vi "Get Counter Updated Event.vi"(8 "error in (no error)":errorcluster, 11 "Counter in":refnum<class "Counter.lvclass">) -> (0 "error out":errorcluster, 2 "Counter Updated":refnum<user-event>, 3 "Counter out":refnum<class "Counter.lvclass">)   [LabVIEW 2018, in "Counter.lvlib" / "Counter.lvclass"]
uses:
  Counter.lvclass
  Counter.lvclass/Counter.ctl
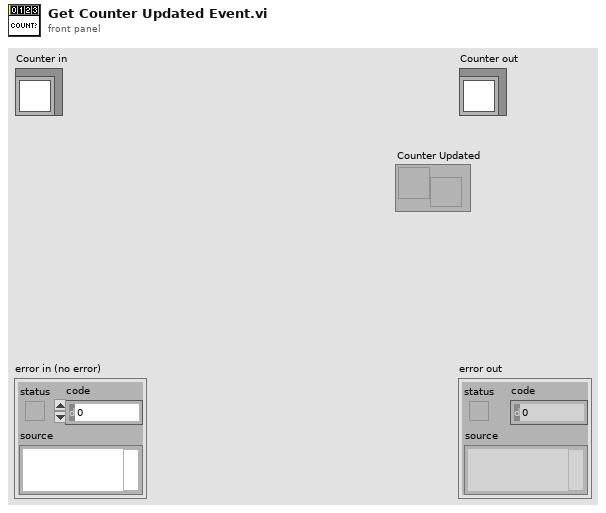
[diagram p1: front panel]
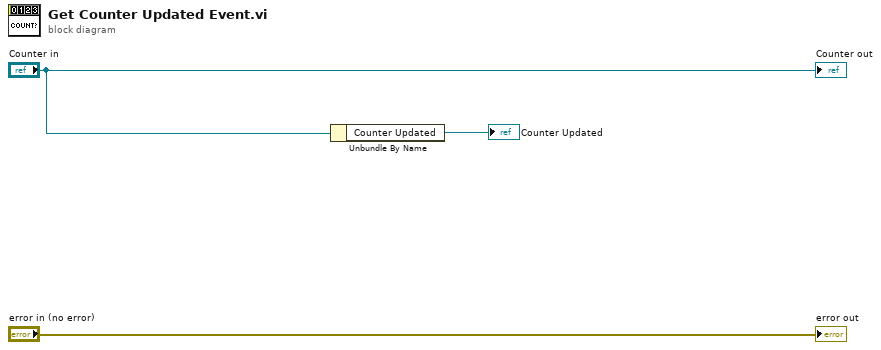
[diagram p0: block diagram]
diagram:
  n1 = Unbundle By Name("Counter in") -> ("Counter Updated"=→"Counter Updated":refnum<user-event>)
  "error out" <- "error in (no error)"
  "Counter out" <- "Counter in"
